vi "Write Mac_Server.vi"(8 "error in (no error)":errorcluster, 10 "Mac/Server":string="9C6B00576F17", 11 "SecureMqttCodec in":refnum<class "SecureMqttCodec.lvclass">) -> (0 "error out":errorcluster, 3 "SecureMqttCodec out":refnum<class "SecureMqttCodec.lvclass">)   [LabVIEW 2020, in "SecureMqttCodec.lvclass"]
uses:
  SecureMqttCodec.lvclass
  SecureMqttCodec.lvclass/SecureMqttCodec.ctl
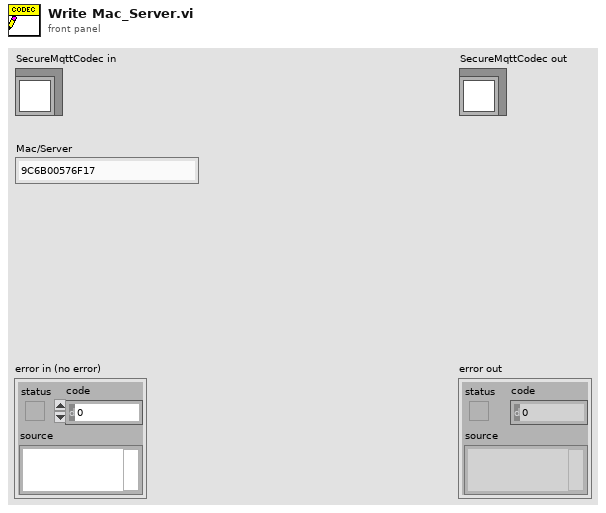
[diagram p1: front panel]
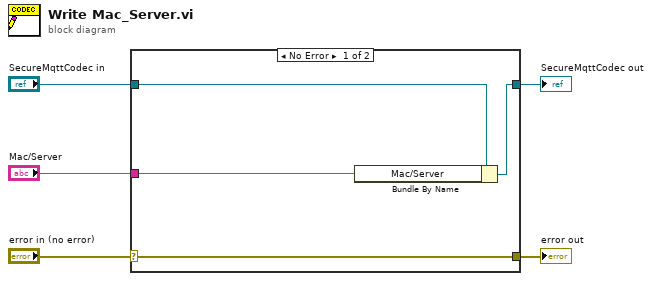
[diagram p0: block diagram]
diagram:
  n1 = case shown="No Error" "error in (no error)" {
    selector: "error in (no error)" -> [w9 w10]
    tunnel: [w9 w10] -> w4
    tunnel: [w7 w11] -> w2
    tunnel: "SecureMqttCodec in" -> [w8 w11]
    tunnel: "Mac/Server" -> [w6 _]
    frame No Error {
      n2 = Bundle By Name(cluster=w8, "Mac/Server"=w6) -> (w7:refnum<class "SecureMqttCodec.lvclass">)
    }
    frame Error {
    }
  }
  "error out" <- w4
  "SecureMqttCodec out" <- w2
